vi "Resample Waveforms.vi"(8 "error in":errorcluster, 11 "PAS Cell Data in":refnum<class "PAS Cell Data.lvclass">) -> (0 "error out":errorcluster, 3 "PAS Cell Data out":refnum<class "PAS Cell Data.lvclass">)   [LabVIEW 2015, in "PAS Cell Data.lvclass"]
doc: "Resampe the waveforms for transmission and display by the host."
uses:
  PAS Cell Data.lvclass
  PAS Cell Data.lvclass/PAS Cell Data.ctl
  <vilib>/Waveform/WDTOps.llb/WDT Get Waveform Subset SGL.vi
  <vilib>/measure/maresamp.llb/Resample Waveform (continuous).vi
  <vilib>/measure/NI_MAPro.lvlib
panel:
  in  "Resample Factor":i32=10
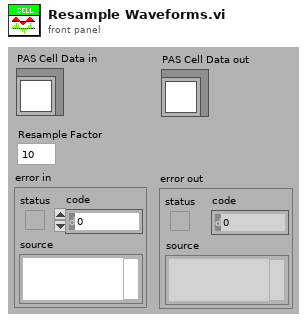
[diagram p1: front panel]
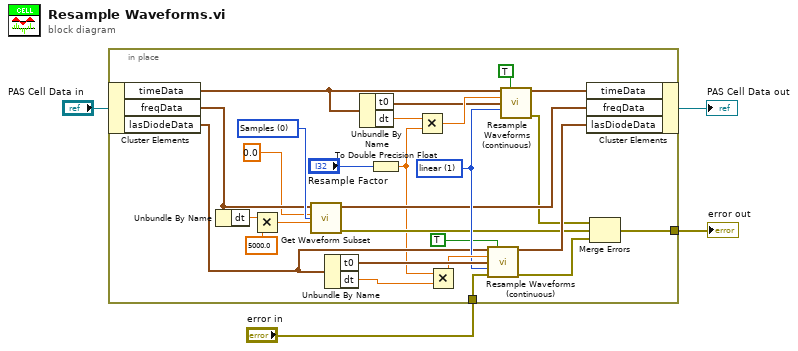
[diagram p0: block diagram]
diagram:
  n1 = in-place {
    in-place-border: [w13] -> w4
    in-place-border: "error in" -> [w9]
    w21 = u16 0 items=["Samples", "Relative Time"] ("start/duration format")
    w22 = u16 1 items=["coerce", "linear", "spline", "FIR filter"] ("interpolation mode")
    n2 = in-place-cluster #1("PAS Cell Data in") -> ("timeData"=w12:waveform(i16), "freqData"=w19:waveform(sgl), "lasDiodeData"=w11:waveform(i16))
    n3 = Unbundle By Name(w19) -> ("dt"=w29:dbl)
    n4 = Multiply(x=w29, y=5000.0) -> (x*y=w30:dbl)
    n5 = call-poly <vilib>:"Get Waveform Subset.vi"("start/duration format"=w21, "duration"=w30, "start samples/time"=0.0, "waveform in"=w19) -> ("error out"=w15:errorcluster, "waveform out"=w18:waveform(sgl))  [unwired: 2 in, 2 out]
    n6 = Unbundle By Name(w11) -> ("t0"=w24:timestamp, "dt"=w6:dbl)
    n7 = Unbundle By Name(w12) -> ("t0"=w25:timestamp, "dt"=w27:dbl)
    n8 = To Double Precision Float(number="Resample Factor") -> (double precision float=w7:dbl)
    n9 = Multiply(x=w27, y=w7) -> (x*y=w26:dbl)
    n10 = Multiply(x=w7, y=w6) -> (x*y=w23:dbl)
    n11 = call-poly <vilib>:"Resample Waveforms (continuous).vi"("waveform in"=w11, "reset"=TRUE, "dt"=w23, "t0"=w24, "interpolation mode"=w22, "error in (no error)"=w9) -> ("resampled waveform out"=w17:waveform(dbl), "error out"=w14:errorcluster)  [unwired: 5 in, 3 out]
    n12 = call-poly <vilib>:"Resample Waveforms (continuous).vi"("waveform in"=w12, "reset"=TRUE, "dt"=w26, "t0"=w25, "interpolation mode"=w22) -> ("resampled waveform out"=w20:waveform(dbl), "error out"=w16:errorcluster)  [unwired: 6 in, 3 out]
    n13 = in-place-cluster #1("timeData"=w20, "freqData"=w18, "lasDiodeData"=w17) -> (→"PAS Cell Data out":refnum<class "PAS Cell Data.lvclass">)
    n14 = Merge Errors(w16, w15, w14) -> (w13:errorcluster)
  }
  "error out" <- w4
